vi "Approach Parametric Position.vi"(4 "Forearm Length":dbl format="%#_13g", 6 "Backarm Length":dbl format="%#_13g", 7 "Points":dbl[][](array[numeric]), 8 "Initial Forearm\nAngle":dbl format="%#_13g", 9 "Initial Backarm\nAngle":dbl format="%#_13g", 10 "Initial Parametric\nValue":dbl format="%#_13g", 11 "New Parametric\nValue":dbl) -> ()   [LabVIEW 2017]
panel:
  out "Next Forearm\nAngle":dbl
  out "Next Backarm\nAngle":dbl
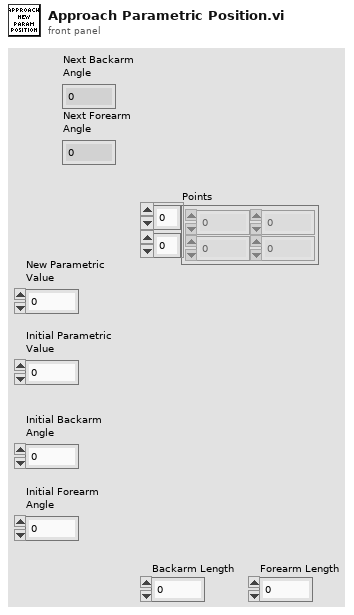
[diagram p1: front panel]
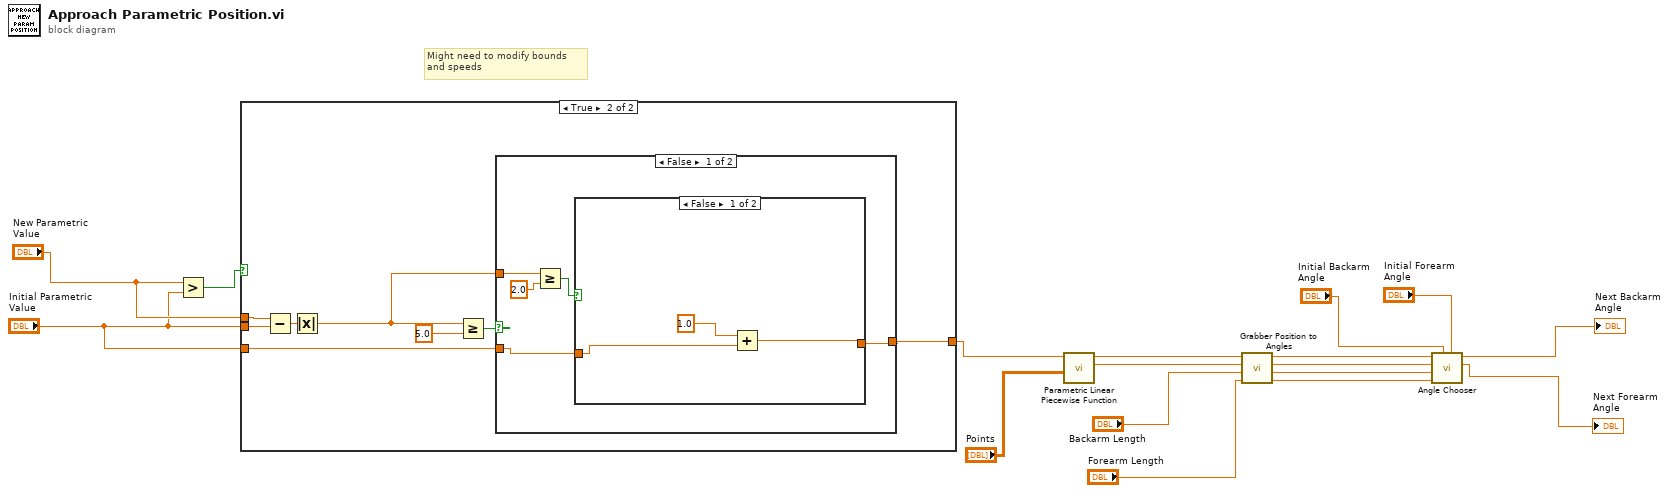
[diagram p0: block diagram]
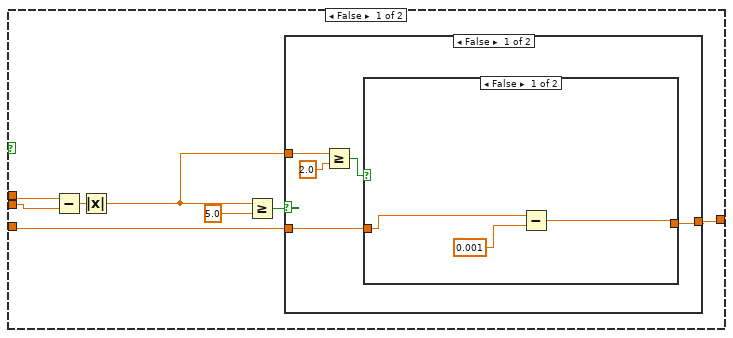
[diagram p2: hidden frame]
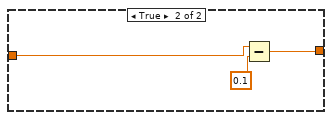
[diagram p3: hidden frame]
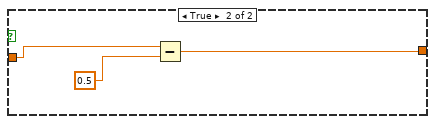
[diagram p4: hidden frame]
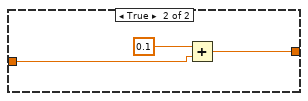
[diagram p5: hidden frame]
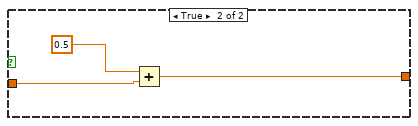
[diagram p6: hidden frame]
diagram:
  # "Might need to modify bounds\nand speeds"
  n1 = Greater?(x="New Parametric\nValue", y="Initial Parametric\nValue") -> (0:w7:bool)
  n2 = case shown="True" w7 {
    tunnel: "Initial Parametric\nValue" -> [w20 w43]
    tunnel: "New Parametric\nValue" -> [w19 w42]
    tunnel: "Initial Parametric\nValue" -> [w21 w41]
    tunnel: [w18 w40] -> w4
    frame False {
      n3 = Subtract(x=w19, y=w20) -> (x-y=w25:dbl)
      n4 = Absolute Value(x=w25) -> (abs(x)=w23:dbl)
      n5 = Greater Or Equal?(x=w23, y=5.0) -> (x >= y?=w24:bool)
      n6 = case shown="False" w24 {
        tunnel: [w27 w37] -> w18
        tunnel: w23 -> [w30 _]
        tunnel: w21 -> [w26 w39]
        frame False {
          n7 = Greater Or Equal?(x=w30, y=2.0) -> (x >= y?=w28:bool)
          n8 = case shown="False" w28 {
            tunnel: [w33 w36] -> w27
            tunnel: w26 -> [w31 w35]
            frame False {
              n9 = Subtract(x=w31, y=0.001 ("x")) -> (x-y=w33:dbl)
            }
            frame True {
              n10 = Subtract(x=w35, y=0.1) -> (x-y=w36:dbl)
            }
          }
        }
        frame True {
          n11 = Subtract(x=w39, y=0.5) -> (x-y=w37:dbl)
        }
      }
    }
    frame True {
      n12 = Subtract(x=w42, y=w43) -> (x-y=w45:dbl)
      n13 = Absolute Value(x=w45) -> (abs(x)=w47:dbl)
      n14 = Greater Or Equal?(x=w47, y=5.0) -> (x >= y?=w46:bool)
      n15 = case shown="False" w46 {
        tunnel: [w49 w61] -> w40
        tunnel: w47 -> [w52 _]
        tunnel: w41 -> [w48 w59]
        frame False {
          n16 = Greater Or Equal?(x=w52, y=2.0) -> (x >= y?=w50:bool)
          n17 = case shown="False" w50 {
            tunnel: [w55 w57] -> w49
            tunnel: w48 -> [w53 w56]
            frame False {
              n18 = Add(x=1.0, y=w53) -> (x+y=w55:dbl)
            }
            frame True {
              n19 = Add(x=0.1, y=w56) -> (x+y=w57:dbl)
            }
          }
        }
        frame True {
          n20 = Add(x=0.5, y=w59) -> (x+y=w61:dbl)
        }
      }
    }
  }
  n21 = call "Parametric Linear Piecewise Function.vi"("Points"="Points", "Parametric\nValue"=w4) -> ("Y Position"=w2:dbl, "X Position"=w1:dbl)  [unwired: 8 in]
  n22 = call "Grabber Position to Angles.vi"("Forearm Length"="Forearm Length", "Backarm Length"="Backarm Length", "Y Initial"=w2, "X Initial"=w1) -> ("Forearm Angle\nDegrees 2"=w14:dbl, "Backarm Angle\nDegrees 2"=w15:dbl, "Forearm Angle\nDegrees 1"=w16:dbl, "Backarm Angle\nDegrees 1"=w17:dbl)  [unwired: 4 in]
  n23 = call "Angle Chooser.vi"("Forearm Angle Initial"="Initial Forearm\nAngle", "Backarm Angle Initial"="Initial Backarm\nAngle", "Forearm Angle 2"=w14, "Backarm Angle 2"=w15, "Forearm Angle 1"=w16, "Backarm Angle 1"=w17) -> ("final Forearm Angle"=→"Next Forearm\nAngle":dbl, "final Backarm Angle"=→"Next Backarm\nAngle":dbl)  [unwired: 4 in]
